vi "SSC DCPower Initiate.vi"(0 "DCPower SSC in":T1[](array[typedef]), 11 "error in":errorcluster) -> (4 "DCPower SSC out":T1[](array[typedef]), 15 "error out":errorcluster)   [LabVIEW 2020]
doc: "Starts generation or acquisition, causing the NI-DCPower sessions to leave the Uncommitted state or Committed state and enter the Running state."
uses:
  SSC DCPower.ctl
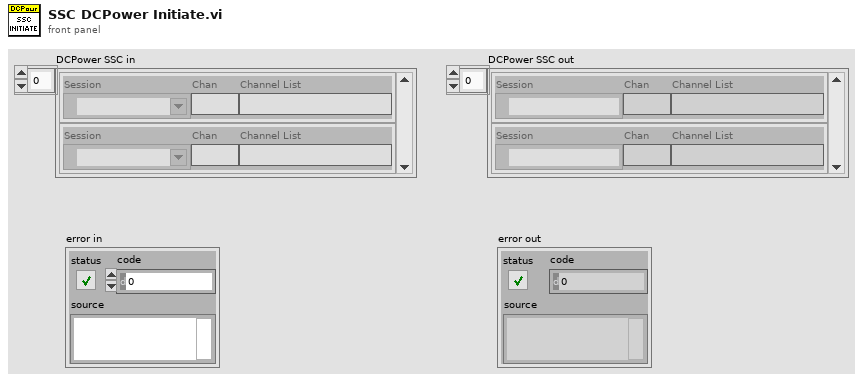
[diagram p1: front panel]
types:
  T1 = typedef "SSC DCPower.ctl" = cluster{"Session":refnum<k15>, "Chan":string, "Channel List":string}
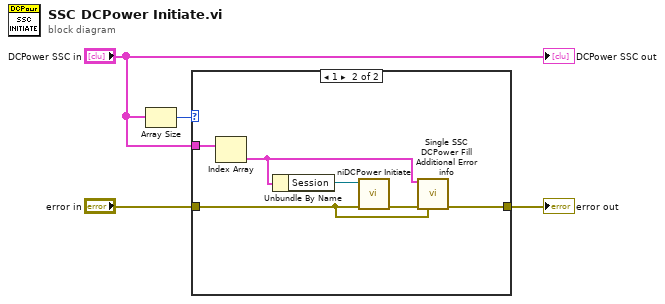
[diagram p0: block diagram]
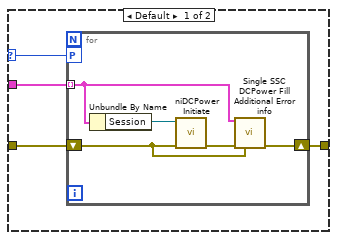
[diagram p2: hidden frame]
diagram:
  n1 = Array Size(array="DCPower SSC in") -> (size(s)=w2:i32)
  n2 = case shown="1" w2 {
    selector: w2 -> [w6 _]
    tunnel: "error in" -> [w8 w19]
    tunnel: [w7 w18] -> w3
    tunnel: "DCPower SSC in" -> [w5 w17]
    frame Default {
      n3 = for {
        tunnel: w5 -> [w10] mode=indexing
        workers-P: w6 -> [_]
        shift-right: [w11] -> w7
        shift-left: w8 -> [w9]
        n4 = Unbundle By Name(w10) -> ("Session"=w12:refnum<k15>)
        n5 = call <instrlib>:"niDCPower Initiate.vi"("error in (no error)"=w9, "instrument handle"=w12) -> ("error out"=w13:errorcluster)  [unwired: 8 in, 1 out]
        n6 = call "Single SSC DCPower Fill Additional Error info.vi"("DCPower SSC in"=w10, "error in"=w13, "previous error in"=w9) -> ("error out"=w11:errorcluster)  [unwired: 12 in]
      }
    }
    frame 1 {
      n7 = Index Array(array=w17) -> (element=w14:T1)  [unwired: 1 in]
      n8 = Unbundle By Name(w14) -> ("Session"=w15:refnum<k15>)
      n9 = call <instrlib>:"niDCPower Initiate.vi"("error in (no error)"=w19, "instrument handle"=w15) -> ("error out"=w16:errorcluster)  [unwired: 8 in, 1 out]
      n10 = call "Single SSC DCPower Fill Additional Error info.vi"("DCPower SSC in"=w14, "error in"=w16, "previous error in"=w19) -> ("error out"=w18:errorcluster)  [unwired: 12 in]
    }
  }
  "error out" <- w3
  "DCPower SSC out" <- "DCPower SSC in"
